vi "Set PID.vi"(8 "error in (no error)":errorcluster, 10 "Control Parameters":cluster{"P":dbl, "I":dbl, "D":u16}[](array[cluster]), 11 "Lakeshore 336 in":refnum<class "Lakeshore 336.lvclass">) -> (0 "error out":errorcluster, 3 "Lakeshore 336 out":refnum<class "Lakeshore 336.lvclass">)   [LabVIEW 2022 SP3, in "Lakeshore 336.lvclass"]
uses:
  Lakeshore 336.lvclass
  Lakeshore 336.lvclass/Lakeshore 336.ctl
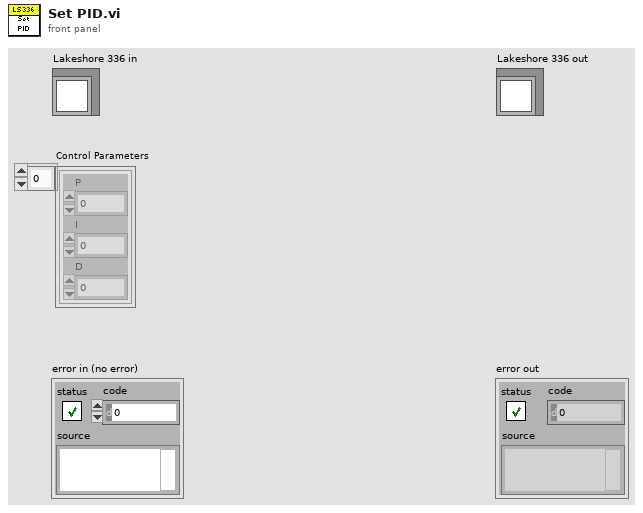
[diagram p1: front panel]
types:
  T1 = typedef "Lakeshore 336.lvclass/Lakeshore 336 Channel Settings cluster.ctl" = cluster{"Input (0:None)":u16, "Power Up Enable (F: Off)":bool, "Mode (0:Off)":u16, "Max Current (0:User Specified)":u16, "Heater Out Display (1:Current)":u16, "Max User Current (2.000)":dbl, "Heater Resistance (1:25 Ohms)":u16, "PID":T2, "Name":string}
  T2 = typedef "Lakeshore 336.lvclass/Lakeshore 336 PID cluster.ctl" = cluster{"P":dbl, "I":dbl, "D":dbl}
  T3 = typedef "Lakeshore 336.lvclass/Lakeshore 336 Settings cluster.ctl" = cluster{"Lake Shore 336 Address":refnum<visa-resource-name>, "Output Ch":T1[], "Input Ch":T4[], "Prefix":string}
  T4 = typedef "Lakeshore 336.lvclass/Lakeshore 336 Input Ch config cluster.ctl" = cluster{"Name":string}
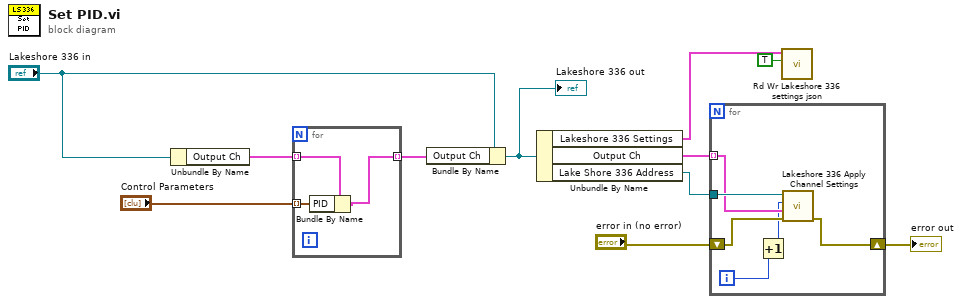
[diagram p0: block diagram]
diagram:
  n1 = Unbundle By Name("Lakeshore 336 in") -> ("Output Ch"=w10:T1[])
  n2 = for {
    tunnel: "Control Parameters" -> [w13] mode=indexing
    tunnel: w10 -> [w14] mode=indexing
    tunnel: [w12] -> w8 mode=indexing
    n3 = Bundle By Name(cluster=w14, "PID"=w13) -> (w12:T1)
  }
  n4 = Bundle By Name(cluster="Lakeshore 336 in", "Output Ch"=w8) -> (w3:refnum<class "Lakeshore 336.lvclass">)
  "Lakeshore 336 out" <- w3
  n5 = Unbundle By Name(w3) -> ("Lakeshore 336 Settings"=w2:T3, "Output Ch"=w7:T1[], "Lake Shore 336 Address"=w6:refnum<visa-resource-name>)
  n6 = for {
    tunnel: w7 -> [w19] mode=indexing
    tunnel: w6 -> [w20]
    shift-right: [w17] -> w4
    shift-left: "error in (no error)" -> [w18]
    i -> [w16]
    n7 = Increment(x=w16) -> (x+1=w15:i32)
    n8 = call "Lakeshore 336 Apply Channel Settings.vi"("error in (no error)"=w18, "Manual Settings"=w19, "Channel (1)"=w15, "Addr"=w20) -> ("error out"=w17:errorcluster)  [unwired: 5 in, 2 out]
  }
  "error out" <- w4
  n9 = call "Rd Wr Lakeshore 336 settings json.vi"("Write? (F:Read)"=TRUE, "Lakeshore 336 Settings"=w2) -> ()  [unwired: 8 in, 2 out]
